vi "EI (B).vi"(0 "Ei":refnum<k24>, 1 "Sampler":refnum<k24>, 2 "Disable Sampler":bool, 5 "error in (no error)":errorcluster) -> (14 "CurrentOverload":bool, 15 "PotentialOverload":bool, 16 "Cell":bool, 17 "ManualCellSwitch":bool, 19 "error out":errorcluster)   [LabVIEW 2011]
doc: "Electrochemical Interface control panel (basic version)"
uses:
  C:/Program Files/Metrohm Autolab/Autolab SDK 1.10/EcoChemie.Autolab.Sdk.dll
  EcoChemie.Autolab.Sdk.dll
panel:
  out "Setpoint":dbl
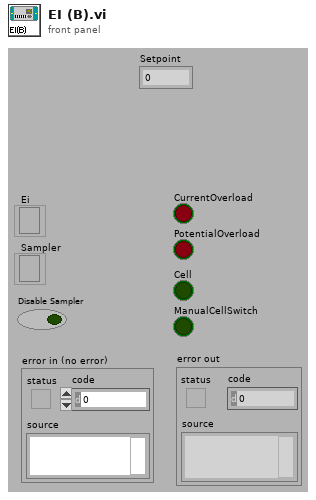
[diagram p1: front panel]
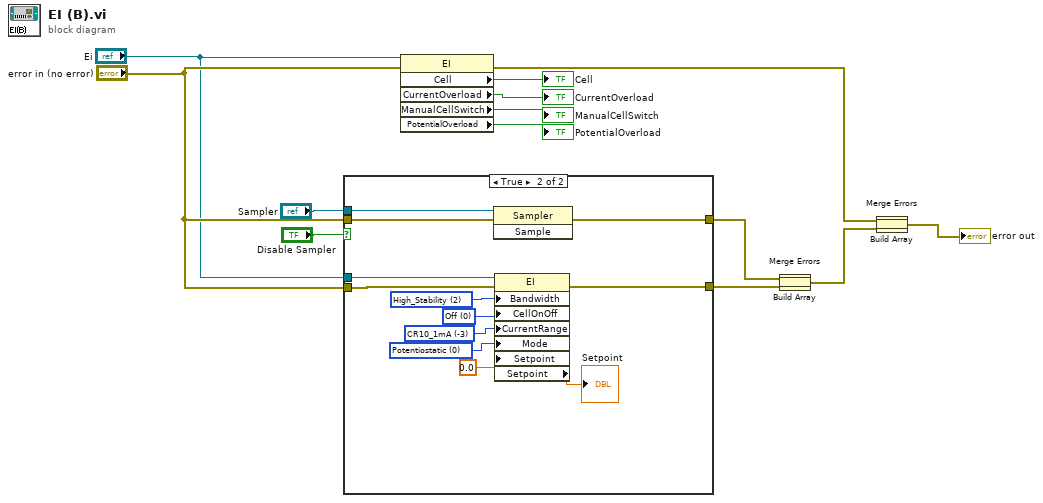
[diagram p0: block diagram]
diagram:
  n1 = case shown="True" "Disable Sampler" {
    tunnel: [w17 w19] -> w9
    tunnel: "error in (no error)" -> [w17 w29]
    tunnel: "Ei" -> [_ w24]
    tunnel: "error in (no error)" -> [w16 w23]
    tunnel: "Sampler" -> [_ w21]
    tunnel: [w16 w20] -> w4
    frame False {
    }
    frame True {
      w25 = 0 items=["Potentiostatic", "Galvanostatic"] ("Mode")
      w26 = -3 items=["CR07_1A"=0, "CR06_10A"=1, "CR01_100A"=2, "CR00_1000A"=3, "CR05_20A"=20, "CR04_40A"=40, "CR03_50A"=60, "CR02_80A"=80, "CR19_1pA"=-12, "CR18_10pA"=-11, "CR17_100pA"=-10, "CR16_1nA"=-9, "CR15_10nA"=-8, "CR14_100nA"=-7, "CR13_1uA"=-6, "CR12_10uA"=-5, "CR11_100uA"=-4, "CR10_1mA"=-3, "CR09_10mA"=-2, "CR08_100mA"=-1] ("CurrentRange")
      w27 = 0 items=["Off", "On"] ("CellOnOff")
      w28 = 2 items=["UltraHigh_Speed", "High_Speed", "High_Stability"] ("Bandwidth")
      n2 = invoke class="Sampler" method="Sample"(reference=w21, error in=w29) -> (error out=w19:errorcluster)  [unwired: 1 in, 2 out]
      n3 = property class="EI"(reference=w24, error in=w23, "Bandwidth"=w28, "CellOnOff"=w27, "CurrentRange"=w26, "Mode"=w25, "Setpoint"=0.0) -> (error out=w20:errorcluster, "Setpoint"=→"Setpoint":dbl)  [unwired: 1 out]
    }
  }
  n4 = property class="EI"(reference="Ei", error in="error in (no error)") -> (error out=w13:errorcluster, "Cell"=→"Cell":bool, "CurrentOverload"=→"CurrentOverload":bool, "ManualCellSwitch"=→"ManualCellSwitch":bool, "PotentialOverload"=→"PotentialOverload":bool)  [unwired: 1 out]
  n5 = Build Array(w9, w4) -> (w2:errorcluster[])
  n6 = Merge Errors(w2) -> (w12:errorcluster)
  n7 = Build Array(w13, w12) -> (w1:errorcluster[])
  n8 = Merge Errors(w1) -> (→"error out":errorcluster)
